vi "String Starts With.vi"(10 "starts with":string, 11 "string":string) -> (2 "starts-with":bool)   [LabVIEW 2020]
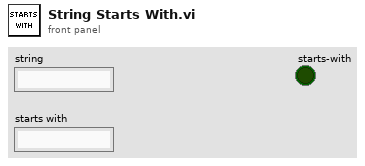
[diagram p1: front panel]
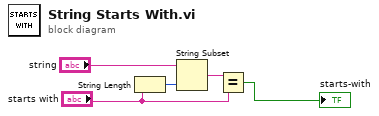
[diagram p0: block diagram]
diagram:
  n1 = String Length(string="starts with") -> (length=w2:i32)
  n2 = String Subset(string="string", length (rest)=w2) -> (substring=w3:string)  [unwired: 1 in]
  n3 = Equal?(x=w3, y="starts with") -> (x = y?=→"starts-with":bool)
